vi "Tbl_Add (SubVI).vi"(10 "meas":string[](array[string]), 11 "Table in":refnum<vi>) -> ()   [LabVIEW 2017]
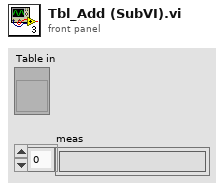
[diagram p1: front panel]
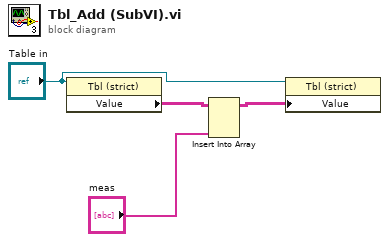
[diagram p0: block diagram]
diagram:
  n1 = property class="Tbl (strict)"(reference="Table in") -> ("Value"=w2:string[][])  [unwired: 1 in, 2 out]
  n2 = Insert Into Array(array=w2, new element="meas") -> (w3:string[][])  [unwired: 2 in]
  n3 = property class="Tbl (strict)"(reference="Table in", "Value"=w3) -> ()  [unwired: 1 in, 2 out]
